vi "HEX TO ASCII.vi"(11 "HEX":string) -> (3 "ASCII":string)   [LabVIEW 2015, in "PLC.lvlib"]
uses:
  PLC.lvlib
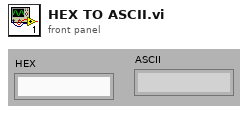
[diagram p1: front panel]
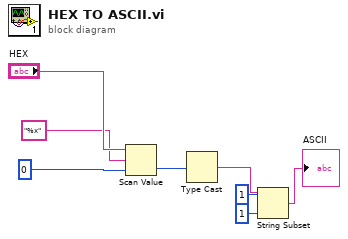
[diagram p0: block diagram]
diagram:
  n1 = Scan Value(string="HEX", format string="%x" ("格式字符串"), default (0 dbl)=i16 0 ("默认(0 dbl)")) -> (value=w5:i16)  [unwired: 1 out]
  n2 = Type Cast(x=w5) -> (*(type *) &x=w4:string)  [unwired: 1 out]
  n3 = String Subset(string=w4, offset (0)=1 ("偏移量(0)"), length (rest)=1 ("长度（剩余）")) -> (substring=→"ASCII":string)
